vi "Xeryon add drive letter.vi"(4 "String in":string, 5 "Drive letter":string) -> (1 "String out":string)   [LabVIEW 2019]
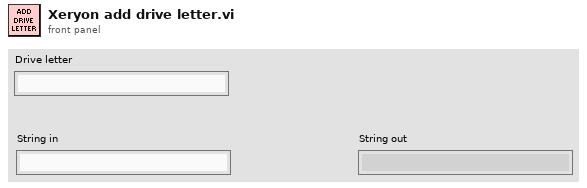
[diagram p1: front panel]
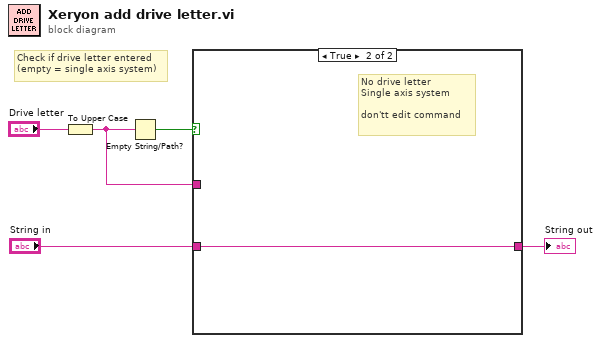
[diagram p0: block diagram]
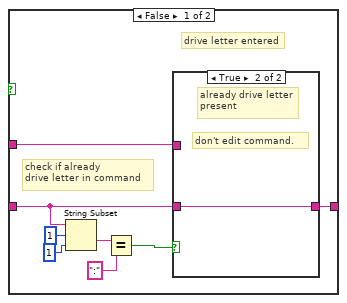
[diagram p2: hidden frame]
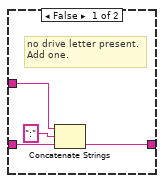
[diagram p3: hidden frame]
diagram:
  # "Check if drive letter entered\n(empty = single axis system)"
  n1 = To Upper Case(1:"Drive letter") -> (0:w1:string)
  n2 = Empty String/Path?(string/path=w1) -> (empty?=w4:bool)
  n3 = case shown="True" w4 {
    tunnel: "String in" -> [w11 w19]
    tunnel: [w13 w19] -> w3
    tunnel: w1 -> [w12 _]
    frame False {
      # "check if already \ndrive letter in command"
      # "drive letter entered"
      n4 = String Subset(string=w11, offset (0)=1, length (rest)=1 ("length (rest)")) -> (substring=w8:string)
      n5 = Equal?(x=w8, y=":") -> (x = y?=w6:bool)
      n6 = case shown="True" w6 {
        tunnel: [w17 w18] -> w13
        tunnel: w12 -> [w16 _]
        tunnel: w11 -> [w14 w18]
        frame False {
          # "no drive letter present.\nAdd one."
          n7 = Concatenate Strings(w16, ":" ("string"), w14) -> (w17:string)
        }
        frame True {
          # "don't edit command."
          # "already drive letter\npresent"
        }
      }
    }
    frame True {
      # "No drive letter\nSingle axis system\n\ndon'tt edit command"
    }
  }
  "String out" <- w3
